vi "Switch alternative path.vi"(8 "error in (no error)":errorcluster, 9 "Alternative path":path, 11 "Original path":path) -> (0 "error out":errorcluster, 1 "Path is empty or does not exist":bool, 3 "Output path":path)   [LabVIEW 2017]
doc: "This VI checks the input folder path (original path). If it is empty or the actual folder does not exist it switches top the alternative path input."
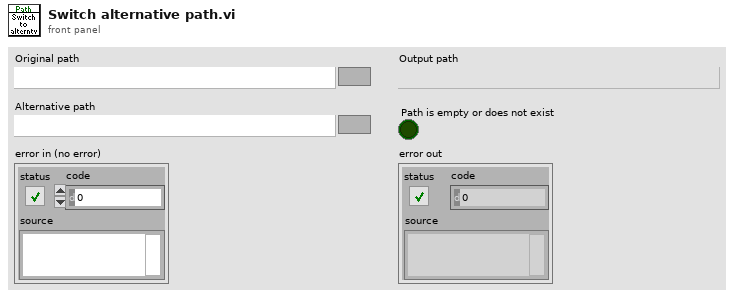
[diagram p1: front panel]
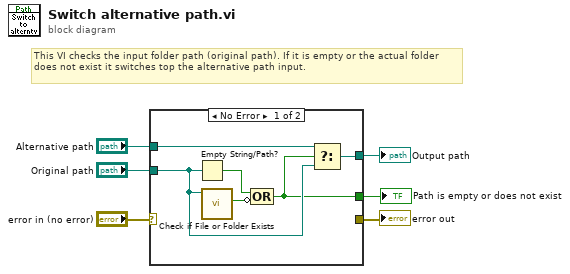
[diagram p0: block diagram]
diagram:
  # "This VI checks the input folder path (original path). If it is empty or the actual folder does not exist it switches top the alternative path input."
  n1 = case shown="No Error" "error in (no error)" {
    selector: "error in (no error)" -> [_ w14]
    tunnel: "Original path" -> [w12 w13]
    tunnel: [w9 w13] -> w5
    tunnel: "Alternative path" -> [w8 _]
    tunnel: [_ w14] -> w2
    tunnel: [w7 _] -> w1
    frame No Error {
      n2 = Empty String/Path?(string/path=w12) -> (empty?=w11:bool)
      n3 = call <vilib>:"Check if File or Folder Exists.vi"("path"=w12) -> ("file or folder exists?"=w10:bool)  [unwired: 8 in, 2 out]
      n4 = Compound Arithmetic op=OR(w11, invert w10) -> (w7:bool)
      n5 = Select(t=w8, s=w7, f=w12) -> (s? t:f=w9:path)
    }
    frame Error {
    }
  }
  "Output path" <- w5
  "error out" <- w2
  "Path is empty or does not exist" <- w1
